vi "Set Value by Query.vi"(8 "error in (no error)":errorcluster, 10 "SQL (use builtin)":string, 11 "Text Column in":refnum<class "Text Column.lvclass">) -> (0 "error out":errorcluster, 3 "Text Column out":refnum<class "Text Column.lvclass">)   [LabVIEW 2020]
uses:
  Text Column.lvclass
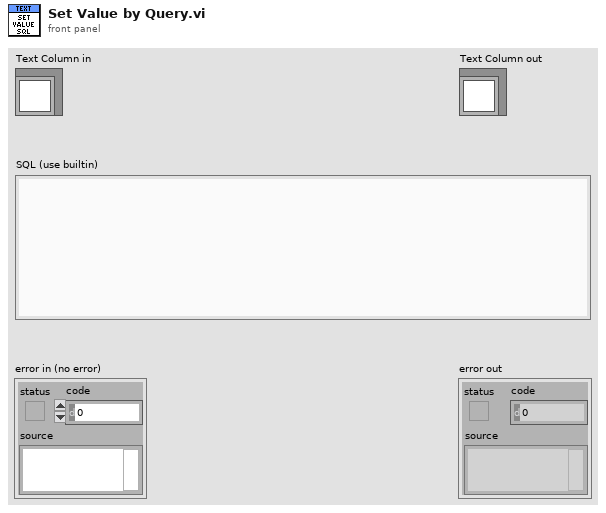
[diagram p1: front panel]
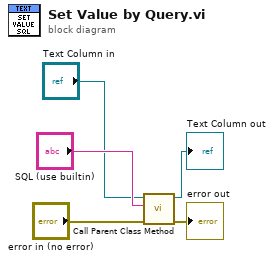
[diagram p0: block diagram]
diagram:
  n1 = call-parent "Call Parent Class Method"("error in (no error)"="error in (no error)", "SQL (use builtin)"="SQL (use builtin)", "Column in"="Text Column in") -> ("error out"=→"error out":errorcluster, "Column out"=→"Text Column out":refnum<class "Text Column.lvclass">)  [unwired: 7 in]
